vi "Set EM Mode and HSS.vi"(8 "error in (no error)":errorcluster, 11 "CCDCamera in":refnum<class "CCDCamera.lvclass">) -> (0 "error out":errorcluster, 3 "CCDCamera out":refnum<class "CCDCamera.lvclass">)   [LabVIEW 2018, in "CCDCamera.lvclass"]
uses:
  CCDCamera.lvclass
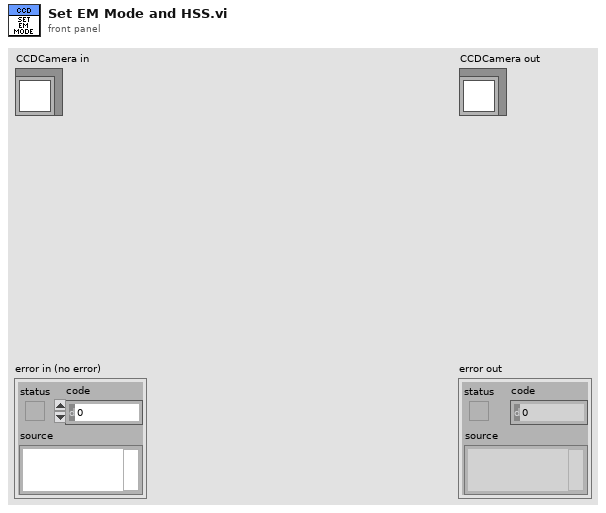
[diagram p1: front panel]
types:
  T1 = cluster{"PREAMP":u16, "READOUT_RATE":u16, "EM_GAIN":u16, "VERTICAL_SHIFT_SPEED":u16, "READ_MODE":u16, "FRAME_TRANSFER":bool, "VERTICAL_CLOCK_VOLTAGE":u16, "ACQUISITION_MODE":u16, "AD_CHANNEL":u16, "EM_MODE":u16, "SHUTTER_TTL":u16, "SHUTTER_OPENING_TIME":u16, "SHUTTER_CLOSING_TIME":u16, "SHUTTER_MODE":u16, "TRIGGER_MODE":u16, "VBIN":u16, "INITIAL_LINE":u16, "INITIAL_COLUMN":u16, "FINAL_LINE":u16, "FINAL_COLUMN":u16, "HBIN":u16}
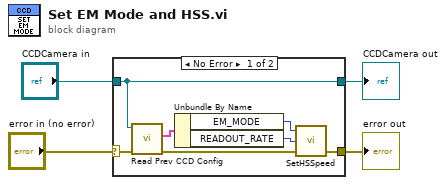
[diagram p0: block diagram]
diagram:
  n1 = case shown="No Error" "error in (no error)" {
    selector: "error in (no error)" -> [w10 w13]
    tunnel: [w11 w13] -> w2
    tunnel: [w5 w12] -> w1
    tunnel: "CCDCamera in" -> [w5 w12]
    frame No Error {
      n2 = call-dynamic "Read Prev CCD Config.vi"("error in (no error)"=w10, "Simulated_CCD_Camera in"=w5) -> ("error out"=w9:errorcluster, "Prev CCD Config"=w8:T1)  [unwired: 7 in, 1 out]
      n3 = Unbundle By Name(w8) -> ("EM_MODE"=w7:u16, "READOUT_RATE"=w6:u16)
      n4 = call <userlib>:"SetHSSpeed.vi"("error in (no error)"=w9, "index"=w6, "type"=w7) -> ("error out"=w11:errorcluster)  [unwired: 1 in, 1 out]
    }
    frame Error {
    }
  }
  "error out" <- w2
  "CCDCamera out" <- w1
